vi "Extract Latest.vi"(8 "Error":errorcluster, 10 "Raw Data Waveform":T1, 11 "(WavIndex_Pointer)":refnum<class "WavIndex_Pointer.lvclass">) -> (0 "Error Out":errorcluster, 2 "Waveform Out":T1, 3 "(WavIndex_Pointer) Out":refnum<class "WavIndex_Pointer.lvclass">)   [LabVIEW 2025, in "WavIndex_Pointer.lvclass"]
uses:
  WavIndex_Pointer.lvclass
  Universal Controls/Waveform_Data.ctl
  WavIndex_Pointer.lvclass/WavIndex_Pointer.ctl
  Index_Pointer/Index_Pointer.lvclass
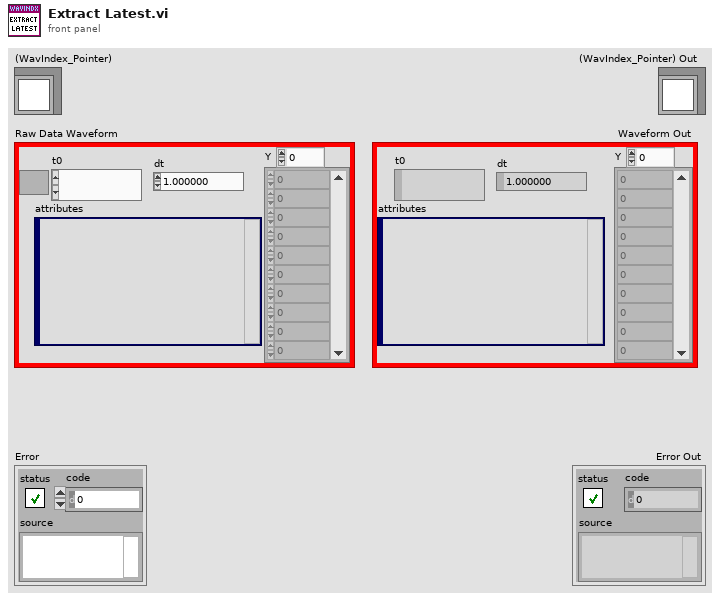
[diagram p1: front panel]
types:
  T1 = typedef "Waveform_Data.ctl" = waveform(dbl)
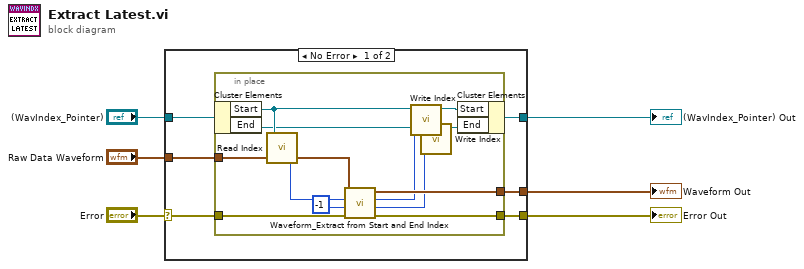
[diagram p0: block diagram]
diagram:
  n1 = case shown="No Error" "Error" {
    selector: "Error" -> [w9 w26]
    tunnel: [w8 w26] -> w5
    tunnel: "Raw Data Waveform" -> [w7 _]
    tunnel: "(WavIndex_Pointer)" -> [w12 w25]
    tunnel: [w11 w25] -> w2
    tunnel: [w10 _] -> w1
    frame No Error {
      n2 = in-place {
        in-place-border: [w24] -> w10
        in-place-border: w9 -> [w23]
        in-place-border: [w22] -> w8
        in-place-border: w7 -> [w13]
        n3 = in-place-cluster #1(w12) -> ("Start"=w20:refnum<class "Index_Pointer.lvclass">, "End"=w17:refnum<class "Index_Pointer.lvclass">)
        n4 = call "Read Index.vi"("Index_Pointer)"=w20) -> ("Index Out"=w21:i32)  [unwired: 2 in]
        n5 = call "Waveform_Extract from Start and End Index.vi"("Error"=w23, "End Index\n(-1) Last point"=-1 ("End Index\n(-1) Last point"), "Start Index"=w21, "Raw Data Waveform"=w13) -> ("Error Out"=w22:errorcluster, "End Out"=w14:i32, "Start Out"=w18:i32, "Waveform Out"=w24:T1)  [unwired: 4 out]
        n6 = call "Write Index.vi"("Index"=w18, "(Index_Pointer) In"=w20) -> ("(Index_Pointer) Out"=w19:refnum<class "Index_Pointer.lvclass">)  [unwired: 9 in]
        n7 = call "Write Index.vi"("Index"=w14, "(Index_Pointer) In"=w17) -> ("(Index_Pointer) Out"=w16:refnum<class "Index_Pointer.lvclass">)  [unwired: 9 in]
        n8 = in-place-cluster #1("Start"=w19, "End"=w16) -> (w11:refnum<class "WavIndex_Pointer.lvclass">)
      }
    }
    frame Error {
    }
  }
  "Error Out" <- w5
  "(WavIndex_Pointer) Out" <- w2
  "Waveform Out" <- w1
